vi "rpc_tsmaster_activate_client.vi"(8 "error in (no error)":errorcluster caption="Incorrect input (no errors)", 9 "AHandle":i32, 10 "AActivate":bool, 11 "Path input":path) -> (0 "error output":errorcluster, 1 "AHandle 2":i32, 2 "return":i32, 3 "Path output":path)   [LabVIEW 2014]
doc: "Function introduction: Activate or deactivate a TSMaster Rpc client\nAfter calling the location to create TSMaster Rpc client\nInput parameter AHHandle: TSMaster Rpc client handle\nAActivate: true=activated, false=deactivated\nReturn value==0: Function execution successful\nOther values: Function execution failed"
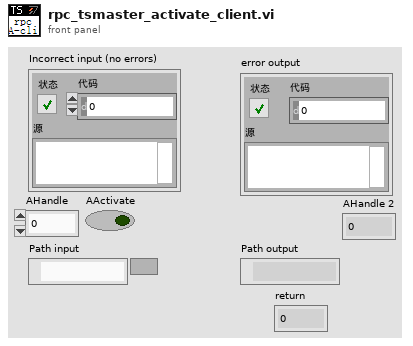
[diagram p1: front panel]
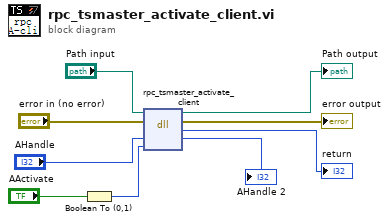
[diagram p0: block diagram]
diagram:
  n1 = Boolean To (0,1)(Boolean="AActivate") -> (0, 1=w2:i16)
  n2 = dll-call lib="C:/Program Files (x86)/TOSUN/TSMaster12/TSMaster/bin/TSMaster.dll" fn="rpc_tsmaster_activate_client"(path in="Path input", error in="error in (no error)", "AHandle"="AHandle", "AActivate"=w2) -> (path out=→"Path output":path, error out=→"error output":errorcluster, "返回类型"=→"return":i32, "AHandle"=→"AHandle 2":i32)  [unwired: 2 in]
